vi "File.Get Folder Differences.vi"(8 "error in (no error)":errorcluster, 9 "Dest Folder":path, 11 "Source Folder":path) -> (0 "error out":errorcluster, 1 "Dest not in Source":path[](array[path]), 2 "Dest":path[](array[path]), 3 "Source":path[](array[path]), 4 "Dest Cnt":i32, 5 "Source Cnt":i32)   [LabVIEW 2024, in "KATE_Lib.lvlib" / "File Utils.lvlib"]
uses:
  File Utils.lvlib
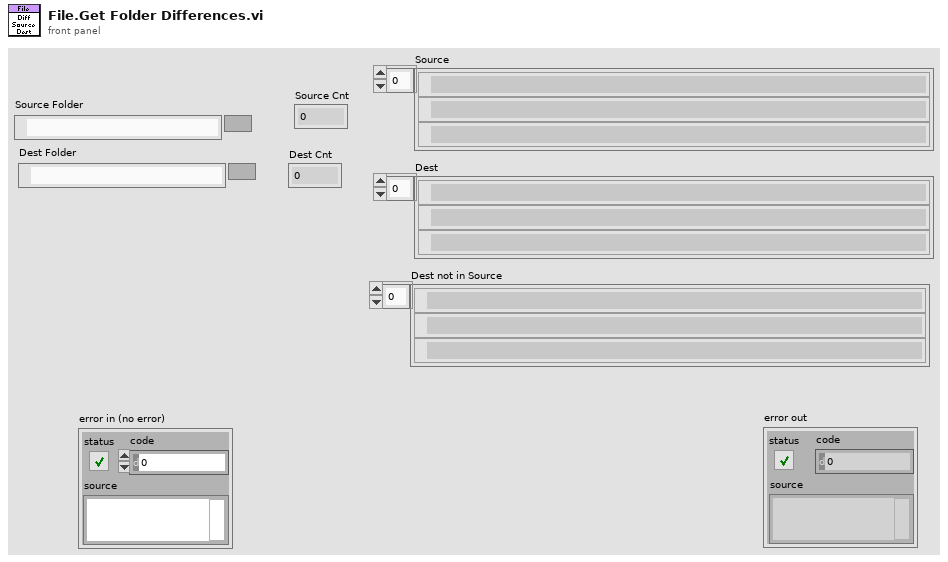
[diagram p1: front panel]
types:
  T1 = typedef "KATE_Lib.lvlib/File Utils.lvlib/File.File Compare Info.ctl" = cluster{"RelPath":string, "path":path, "size":i64, "LastMod":timestamp}
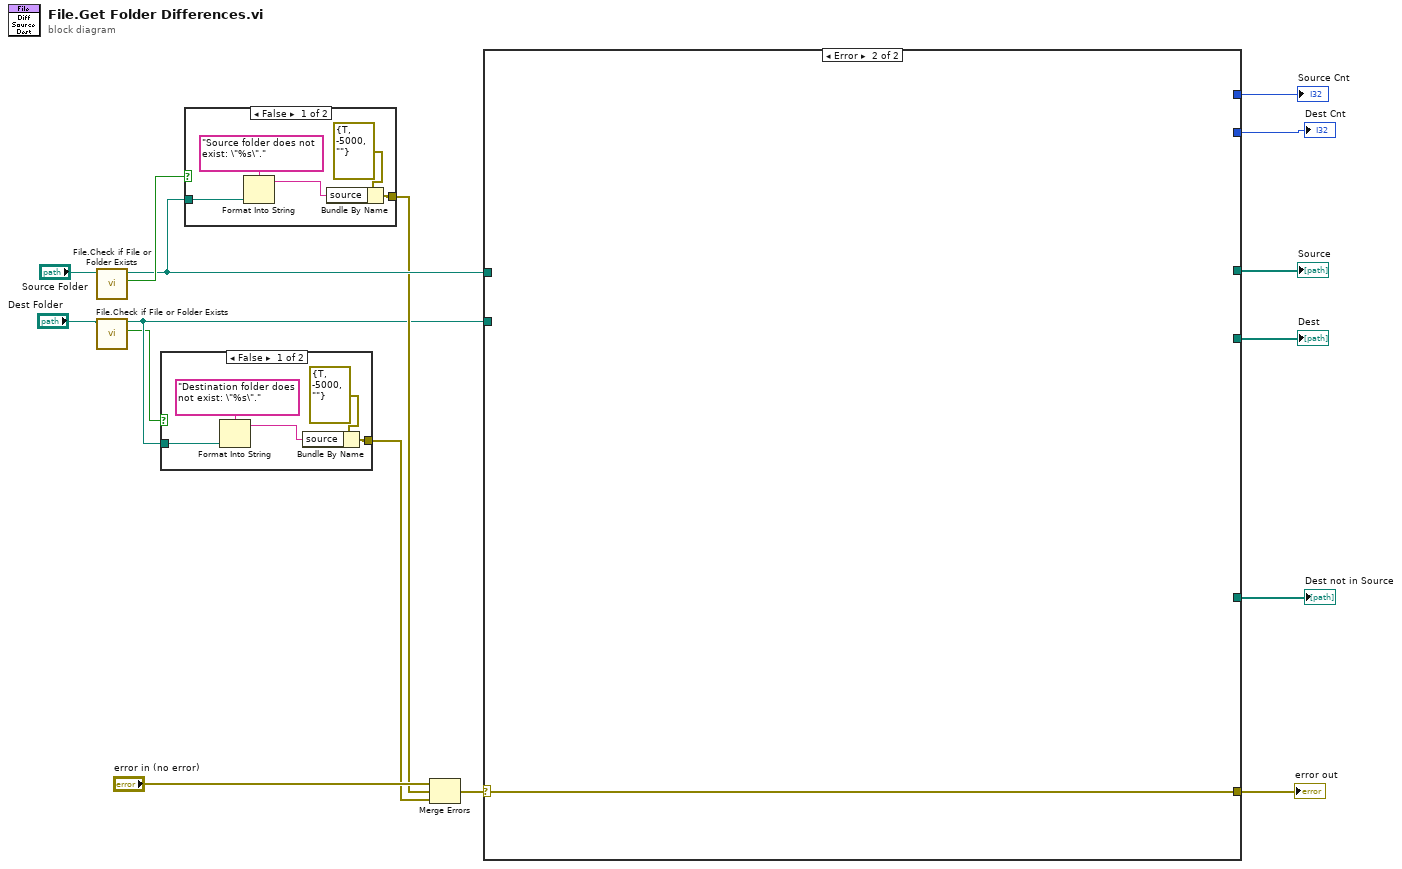
[diagram p0: block diagram]
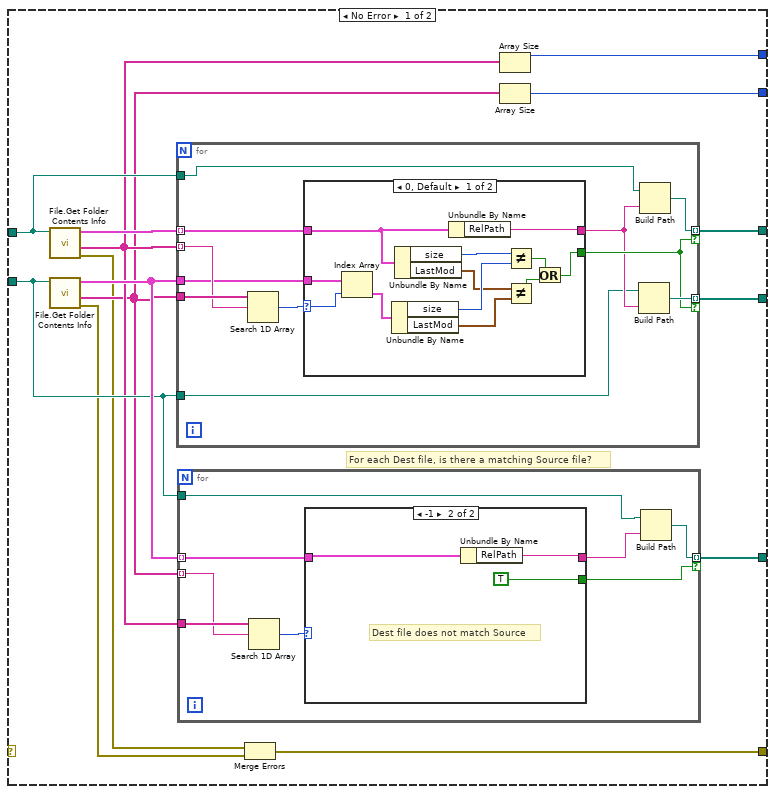
[diagram p4: hidden frame]
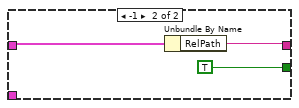
[diagram p6: hidden frame]
diagram:
  n1 = call "File.Check if File or Folder Exists.vi"("Path"="Source Folder") -> ("Exists"=w6:bool, "Dup Path"=w5:path)  [unwired: 6 in, 3 out]
  n2 = call "File.Check if File or Folder Exists.vi"("Path"="Dest Folder") -> ("Exists"=w2:bool, "Dup Path"=w3:path)  [unwired: 6 in, 3 out]
  n3 = case shown="False" w2 {
    tunnel: w3 -> [w20 _]
    tunnel: [w17 _] -> w1
    frame False {
      n4 = Format Into String(format string="Destination folder does not exist: \"%s\".", w20) -> (resulting string=w18:string)  [unwired: 2 in, 1 out]
      n5 = Bundle By Name(cluster=errorcluster {"status"=TRUE, "code"=-5000, "source"=""} ("error constant"), "source"=w18) -> (w17:errorcluster)
    }
    frame True {
    }
  }
  n6 = case shown="False" w6 {
    tunnel: w5 -> [w25 _]
    tunnel: [w22 _] -> w4
    frame False {
      n7 = Format Into String(format string="Source folder does not exist: \"%s\".", w25) -> (resulting string=w23:string)  [unwired: 2 in, 1 out]
      n8 = Bundle By Name(cluster=errorcluster {"status"=TRUE, "code"=-5000, "source"=""} ("error constant"), "source"=w23) -> (w22:errorcluster)
    }
    frame True {
    }
  }
  n9 = Merge Errors("error in (no error)", w4, w1) -> (w8:errorcluster)
  n10 = case shown="Error" w8 {
    selector: w8 -> [_ w78]
    tunnel: w5 -> [w40 _]
    tunnel: [w39 _] -> w16
    tunnel: [w38 _] -> w15
    tunnel: w3 -> [w35 _]
    tunnel: [w34 _] -> w14
    tunnel: [w31 _] -> w13
    tunnel: [w30 _] -> w12
    tunnel: [w27 w78] -> w11
    frame No Error {
      # "For each Dest file, is there a matching Source file?"
      n11 = call "File.Get Folder Contents Info.vi"("Folder"=w40) -> ("error out"=w29:errorcluster, "RelPaths"=w33:string[], "File Info"=w37:T1[])  [unwired: 8 in]
      n12 = call "File.Get Folder Contents Info.vi"("Folder"=w35) -> ("error out"=w28:errorcluster, "RelPaths"=w32:string[], "File Info"=w36:T1[])  [unwired: 8 in]
      n13 = for {
        tunnel: w37 -> [w59] mode=indexing
        tunnel: w36 -> [w58]
        tunnel: w33 -> [w61] mode=indexing
        tunnel: w32 -> [w62]
        tunnel: [w57] -> w39 mode=indexing if=w55
        tunnel: [w56] -> w38 mode=indexing if=w55
        tunnel: w40 -> [w53]
        tunnel: w35 -> [w52]
        n14 = Search 1D Array(1D array=w62, element=w61) -> (index of element=w60:i32)  [unwired: 1 in]
        n15 = case shown="0, Default" w60 {
          selector: w60 -> [w73 _]
          tunnel: w59 -> [w64 w76]
          tunnel: [w63 w75] -> w54
          tunnel: [w65 TRUE] -> w55
          tunnel: w58 -> [w74 _]
          frame 0, Default {
            n16 = Index Array(array=w74, index=w73) -> (element=w72:T1)
            n17 = Unbundle By Name(w72) -> ("size"=w70:i64, "LastMod"=w68:timestamp)
            n18 = Unbundle By Name(w64) -> ("size"=w71:i64, "LastMod"=w69:timestamp)
            n19 = Unbundle By Name(w64) -> ("RelPath"=w63:string)
            n20 = Not Equal?(x=w71, y=w70) -> (x != y?=w67:bool)
            n21 = Not Equal?(x=w69, y=w68) -> (x != y?=w66:bool)
            n22 = Or(x=w67, y=w66) -> (x .or. y?=w65:bool)
          }
          frame -1 {
            n23 = Unbundle By Name(w76) -> ("RelPath"=w75:string)
          }
        }
        n24 = Build Path(base path=w52, name or relative path=w54) -> (appended path=w56:path)
        n25 = Build Path(base path=w53, name or relative path=w54) -> (appended path=w57:path)
      }
      n26 = for {
        tunnel: w36 -> [w45] mode=indexing
        tunnel: w32 -> [w47] mode=indexing
        tunnel: w33 -> [w48]
        tunnel: [w44] -> w34 mode=indexing if=w43
        tunnel: w35 -> [w41]
        n27 = Search 1D Array(1D array=w48, element=w47) -> (index of element=w46:i32)  [unwired: 1 in]
        n28 = case shown="-1" w46 {
          tunnel: w45 -> [_ w50]
          tunnel: [_ w49] -> w42
          tunnel: [_ TRUE] -> w43
          frame 0, Default {
          }
          frame -1 {
            # "Dest file does not match Source"
            n29 = Unbundle By Name(w50) -> ("RelPath"=w49:string)
          }
        }
        n30 = Build Path(base path=w41, name or relative path=w42) -> (appended path=w44:path)
      }
      n31 = Merge Errors(w29, w28) -> (w27:errorcluster)
      n32 = Array Size(array=w33) -> (size(s)=w30:i32)
      n33 = Array Size(array=w32) -> (size(s)=w31:i32)
    }
    frame Error {
    }
  }
  "Source" <- w16
  "Dest" <- w15
  "Dest not in Source" <- w14
  "Source Cnt" <- w12
  "Dest Cnt" <- w13
  "error out" <- w11
